vi "AuthVerifyConnectionInfoResponse_Parse.vi"(8 "error in (no error)":errorcluster, 11 "Message":T5) -> (0 "error out":errorcluster, 1 "Body":T1, 2 "Header":T3, 3 "AuthVerifyConnectionInfoResponse":T2)   [LabVIEW 2017]
uses:
  <vilib>/addons/InsightCM/MessageBus/Base/controls/Message.ctl
  <vilib>/addons/InsightCM/MessageBus/Base/controls/MessageHeader.ctl
  <vilib>/addons/InsightCM/MessageBus/Base/controls/KeyValuePair.ctl
  <vilib>/addons/InsightCM/MessageBus/MessageLibrary/Authentication/controls/AuthVerifyConnectionInfoResponse.ctl
  <vilib>/addons/InsightCM/MessageBus/MessageLibrary/Authentication/controls/AuthVerifyConnectionInfoResponseBody.ctl
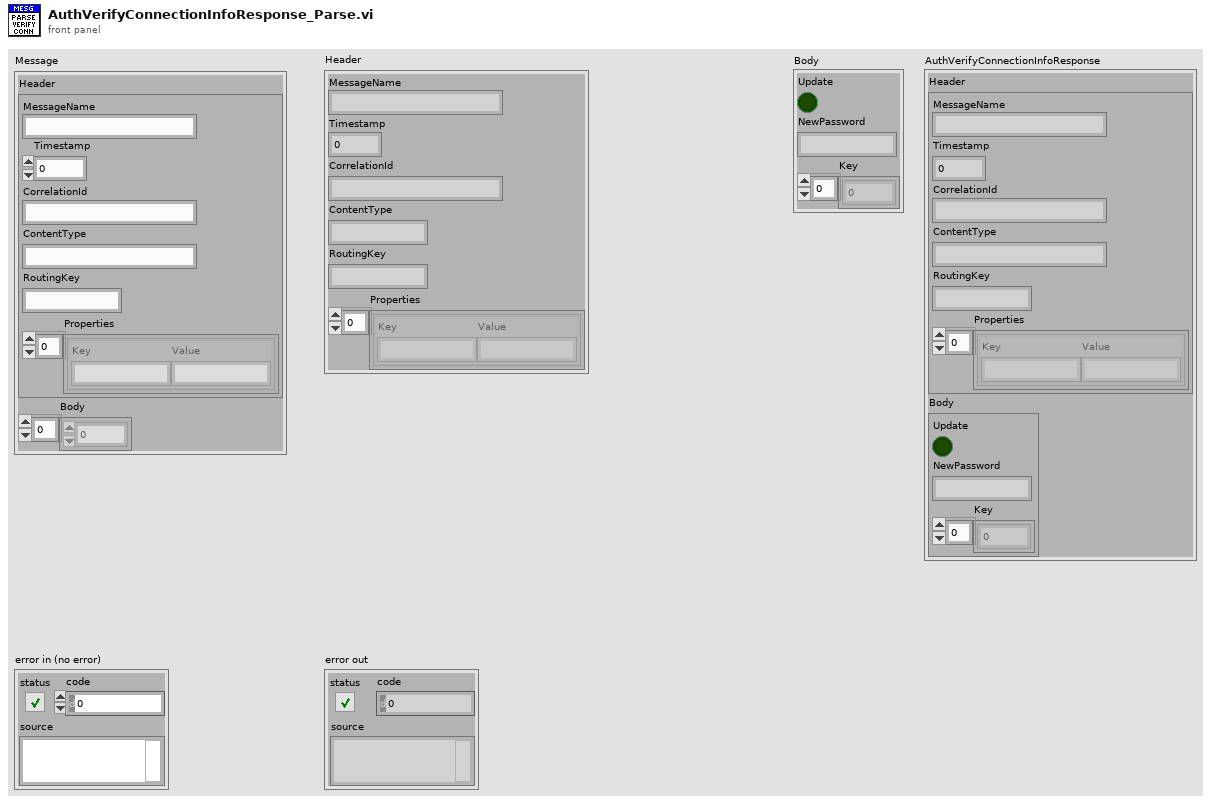
[diagram p1: front panel]
types:
  T1 = typedef "AuthVerifyConnectionInfoResponseBody.ctl" = cluster{"Update":bool, "NewPassword":string, "Key":u8[]}
  T2 = typedef "AuthVerifyConnectionInfoResponse.ctl" = cluster{"Header":T3, "Body":T1}
  T3 = typedef "MessageHeader.ctl" = cluster{"MessageName":string, "Timestamp":i64, "CorrelationId":string, "ContentType":string, "RoutingKey":string, "Properties":T4[]}
  T4 = typedef "KeyValuePair.ctl" = cluster{"Key":string, "Value":string}
  T5 = typedef "Message.ctl" = cluster{"Header":T3, "Body":u8[]}
  T6 = cluster{"Update":bool, "NewPassword":string, "Key":string}
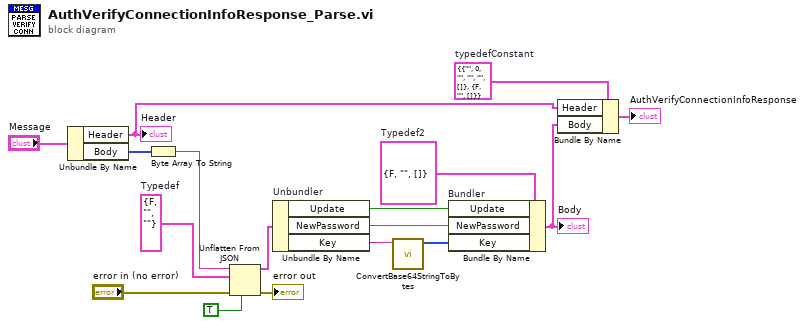
[diagram p0: block diagram]
diagram:
  w5 = T1 {"Update"=FALSE, "NewPassword"="", "Key"=[]}  # Typedef2
  w9 = T2 {"Header"={"MessageName"="", "Timestamp"=0, "CorrelationId"="", "ContentType"="", "RoutingKey"="", "Properties"=[]}, "Body"={"Update"=FALSE, "NewPassword"="", "Key"=[]}}  # typedefConstant
  w13 = T6 {"Update"=FALSE, "NewPassword"="", "Key"=""}  # Typedef
  n1 = Unbundle By Name("Message") -> ("Header"=w15:T3, "Body"=w7:u8[])
  "Header" <- w15
  n2 = Byte Array To String(unsigned byte array=w7) -> (string=w12:string)
  n3 = Unflatten From JSON(JSON string=w12, type and defaults=w13, default null elements? (F)=TRUE, error in (no error)="error in (no error)") -> (value=w11:T6, error out=→"error out":errorcluster)  [unwired: 3 in]
  n4 = Unbundle By Name "Unbundler"(w11) -> ("Update"=w4:bool, "NewPassword"=w3:string, "Key"=w2:string)
  n5 = call <vilib>:"ConvertBase64StringToBytes.vi"("Base64 string"=w2) -> ("U8 array"=w1:u8[])  [unwired: 9 in, 1 out]
  n6 = Bundle By Name "Bundler"(cluster=w5, "Update"=w4, "NewPassword"=w3, "Key"=w1) -> (w6:T1)
  "Body" <- w6
  n7 = Bundle By Name(cluster=w9, "Header"=w15, "Body"=w6) -> (→"AuthVerifyConnectionInfoResponse":T2)
